vi "Part 2.vi"(11 "Input":string) -> (3 "Output":i64)   [LabVIEW 2021]
uses:
  ffae0918-5da2-4e65-addf-7a6bd5d7737e.vi
  <userlib>/_OpenG.lib/string/string.llb/Convert EOLs (String)__ogtk.vi
panel:
  out "XY Graph":cluster{"X":i32, "Y":i32}[](graph)
  out "array":string[](array[string])
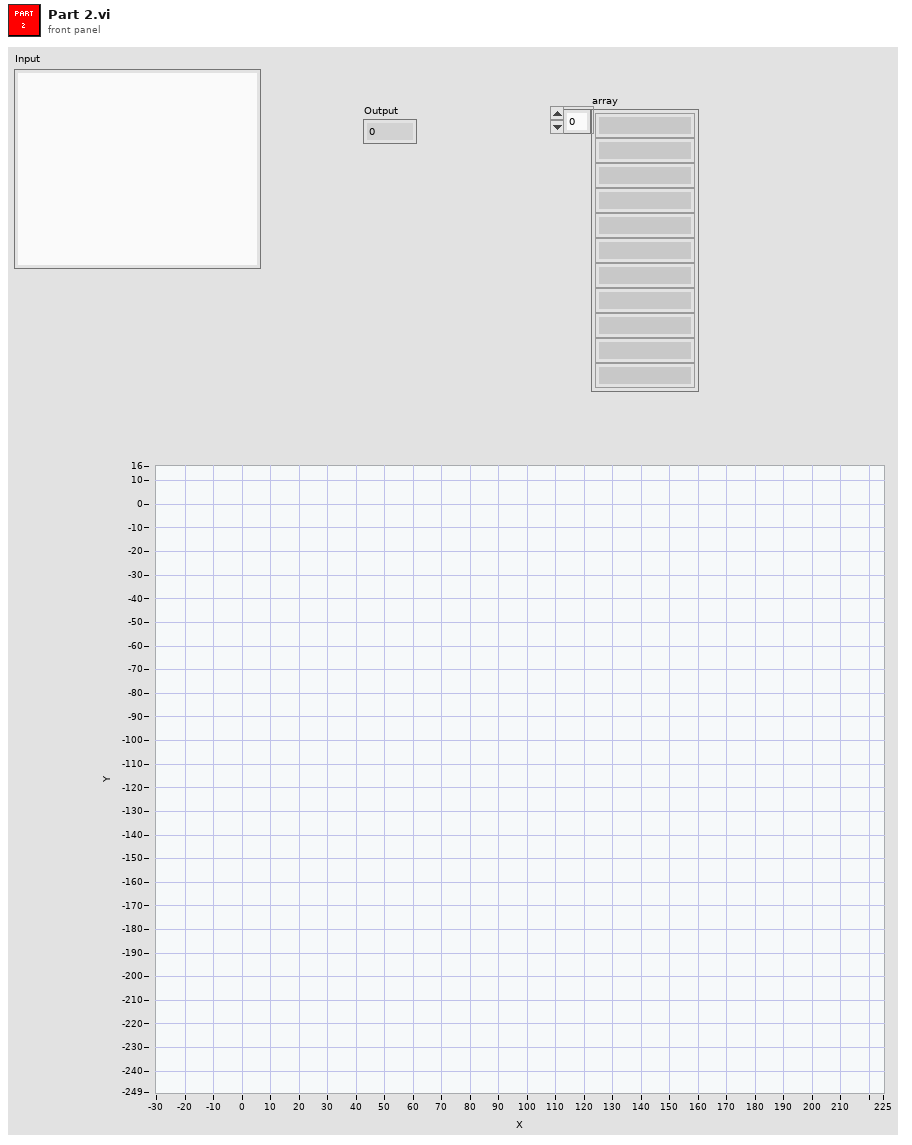
[diagram p1: front panel]
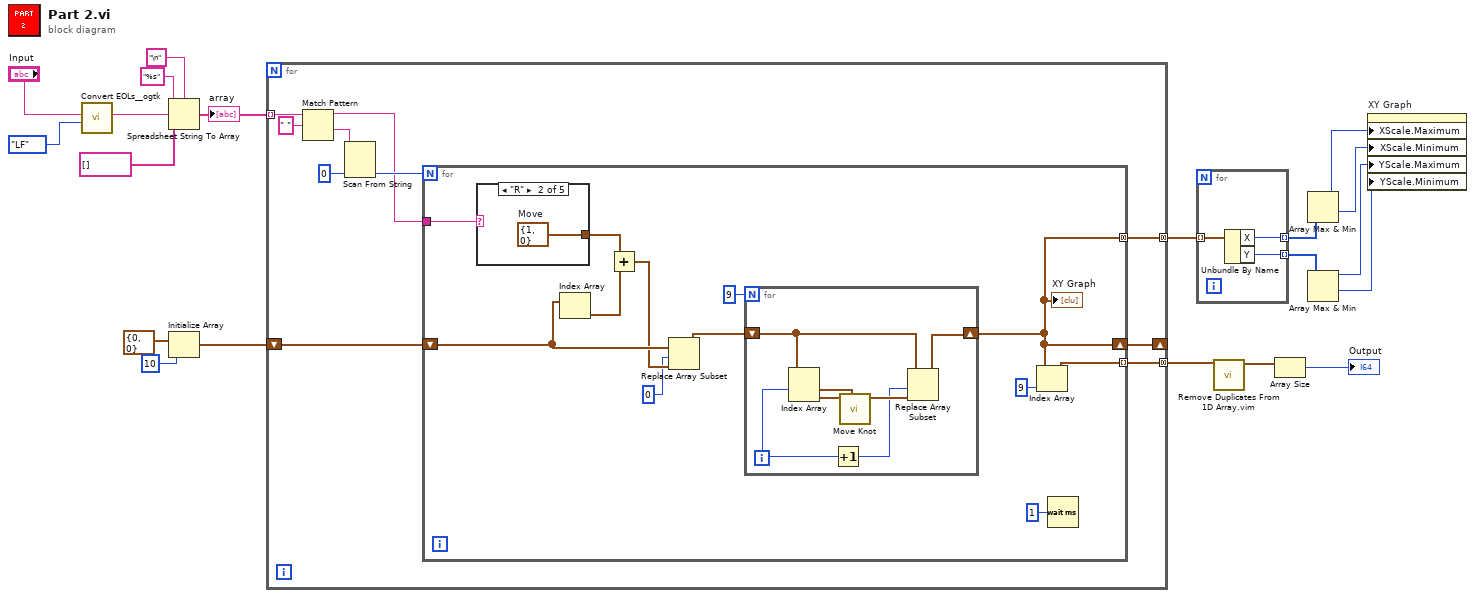
[diagram p0: block diagram]
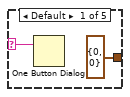
[diagram p2: hidden frame]
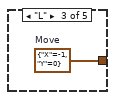
[diagram p3: hidden frame]
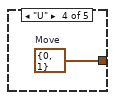
[diagram p4: hidden frame]
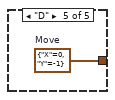
[diagram p5: hidden frame]
diagram:
  n1 = call-poly <userlib>:"Convert EOLs__ogtk.vi"("Convert to:"=enum16{"CR", "LF", "CRLF"}."LF", "String in"="Input") -> ("String out"=w17:string)  [unwired: 9 in]
  n2 = Spreadsheet String To Array(delimiter (Tab)="\n", format string="%s", spreadsheet string=w17, array type (2D Dbl)=string[] []) -> (array=w15:string[])
  "array" <- w15
  n3 = Initialize Array(cluster{"X":i32, "Y":i32} {"X"=0, "Y"=0} ("Tail Pos"), 10 ("dimension size")) -> (w8:cluster{"X":i32, "Y":i32}[])
  n4 = for {
    tunnel: w15 -> [w30] mode=indexing
    shift-right: [w23] -> _
    shift-left: w8 -> [w25]
    tunnel: [w22] -> w14 mode=concatenating
    tunnel: [w21] -> w7 mode=concatenating
    n5 = Match Pattern(string=w30, regular expression=" ") -> (before substring=w24:string, after substring=w28:string)  [unwired: 1 in, 2 out]
    n6 = Scan From String(input string=w28, default 1=0) -> (output 1=w26:i32)  [unwired: 3 in, 3 out]
    n7 = for {
      N: w26 -> [_]
      shift-right: [w31] -> w23
      shift-left: w25 -> [w36]
      tunnel: w24 -> [w42]
      tunnel: [w39] -> w22 mode=indexing
      tunnel: [w31] -> w21 mode=concatenating
      n8 = case shown="\"R\"" w42 {
        selector: w42 -> [w51 _ _ _ _]
        tunnel: [cluster{"X":i32, "Y":i32} {"X"=0, "Y"=0} ("Move") w52 w53 w54 w55] -> w41
        frame Default {
          n9 = One Button Dialog(message=w51) -> ()  [unwired: 1 in, 1 out]
        }
        frame "R" {
          w52 = cluster{"X":i32, "Y":i32} {"X"=1, "Y"=0}  # Move
        }
        frame "L" {
          w53 = cluster{"X":i32, "Y":i32} {"X"=-1, "Y"=0}  # Move
        }
        frame "U" {
          w54 = cluster{"X":i32, "Y":i32} {"X"=0, "Y"=1}  # Move
        }
        frame "D" {
          w55 = cluster{"X":i32, "Y":i32} {"X"=0, "Y"=-1}  # Move
        }
      }
      n10 = Index Array(array=w36) -> (element=w37:cluster{"X":i32, "Y":i32})  [unwired: 1 in]
      n11 = Add(x=w41, y=w37) -> (x+y=w35:cluster{"X":i32, "Y":i32})
      n12 = Replace Array Subset(array=w36, new element=w35, index=0) -> (w34:cluster{"X":i32, "Y":i32}[])
      n13 = for {
        N: 9 -> [_]
        shift-right: [w46] -> w31
        shift-left: w34 -> [w47]
        i -> [w44]
        n14 = Index Array(array=w47, index #1=w44) -> (element #1=w48:cluster{"X":i32, "Y":i32}, element #2=w49:cluster{"X":i32, "Y":i32})  [unwired: 1 in]
        n15 = Increment(x=w44) -> (x+1=w43:i32)
        n16 = call "Move Knot.vi"("Previous knot"=w48, "Current Knot In"=w49) -> ("Current Knot Out"=w45:cluster{"X":i32, "Y":i32})  [unwired: 9 in]
        n17 = Replace Array Subset(array=w47, new element=w45, index=w43) -> (w46:cluster{"X":i32, "Y":i32}[])
      }
      "XY Graph" <- w31
      n18 = Index Array(array=w31, index=9) -> (element=w39:cluster{"X":i32, "Y":i32})
      n19 = Wait (ms)(milliseconds to wait=u32 1) -> ()  [unwired: 1 out]
    }
  }
  n20 = for {
    tunnel: w7 -> [w58] mode=indexing
    tunnel: [w57] -> w6 mode=indexing
    tunnel: [w56] -> w5 mode=indexing
    n21 = Unbundle By Name(w58) -> ("X"=w57:i32, "Y"=w56:i32)
  }
  n22 = call "Remove Duplicates From 1D Array.vim"("array"=w14) -> ("array with duplicates removed"=w13:cluster{"X":i32, "Y":i32}[])  [unwired: 10 in]
  n23 = Array Size(array=w13) -> (size(s)=→"Output":i32)
  n24 = Array Max & Min(array=w6) -> (max value=w4:i32, min value=w3:i32)  [unwired: 2 out]
  n25 = Array Max & Min(array=w5) -> (max value=w2:i32, min value=w1:i32)  [unwired: 2 out]
  n26 = property on="XY Graph" class="XYGraph (strict)"("XScale.Maximum"=w4, "XScale.Minimum"=w3, "YScale.Maximum"=w2, "YScale.Minimum"=w1) -> ()  [unwired: 2 in, 2 out]
